vi "svl_Check Integration Time.vi"(4 "integration time":dbl=1.0 format="%.2f", 6 "acquisition period":dbl=1.0 format="%.2f", 8 "error in (no error)":errorcluster, 9 "restart averaging (F)":bool) -> (0 "error out":errorcluster, 1 "blocks to integrate":i32=1, 2 "parameter has changed":bool)   [LabVIEW 2017]
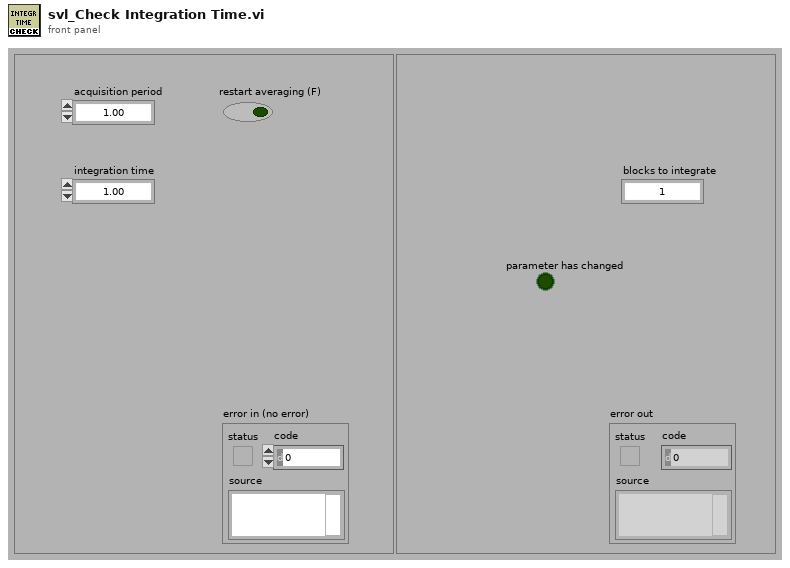
[diagram p1: front panel]
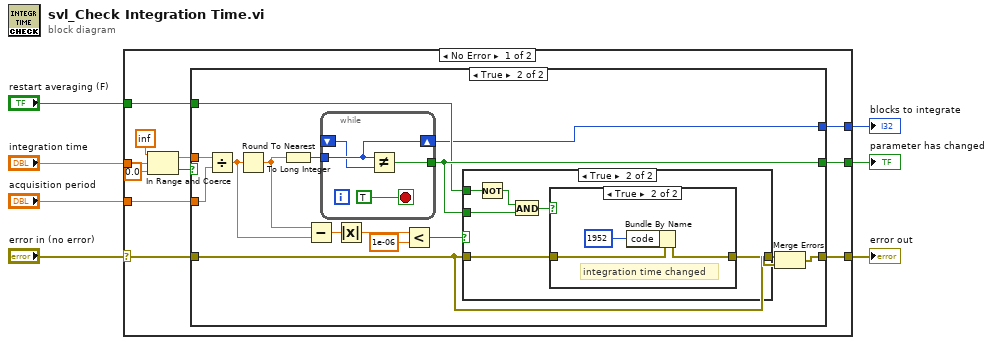
[diagram p0: block diagram]
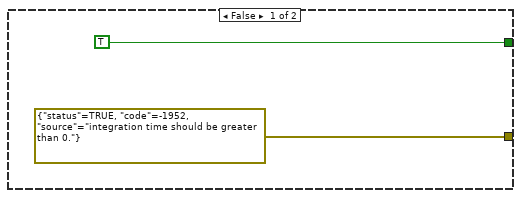
[diagram p2: hidden frame]
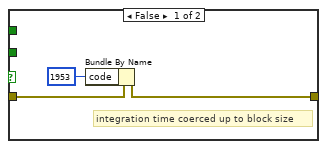
[diagram p3: hidden frame]
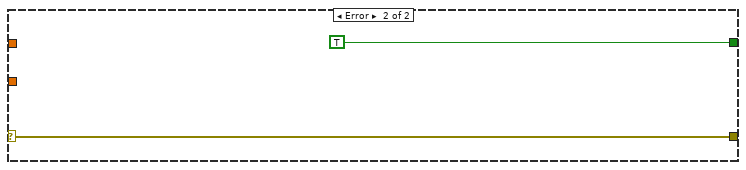
[diagram p5: hidden frame]
diagram:
  n1 = case shown="No Error" "error in (no error)" {
    selector: "error in (no error)" -> [w17 w53]
    tunnel: [w18 TRUE] -> w4
    tunnel: "integration time" -> [w14 _]
    tunnel: [w16 w53] -> w5
    tunnel: "acquisition period" -> [w15 _]
    tunnel: "restart averaging (F)" -> [w9 _]
    tunnel: [w8 _] -> w1
    frame No Error {
      n2 = In Range and Coerce(upper limit=inf, x=w14, lower limit=0.0) -> (coerced(x)=w13:dbl, In Range?=w10:bool)
      n3 = case shown="True" w10 {
        tunnel: [TRUE w35] -> w18
        tunnel: w13 -> [_ w34]
        tunnel: w17 -> [_ w21]
        tunnel: [errorcluster {"status"=TRUE, "code"=-1952, "source"="integration time should be greater than 0."} ("error IO") w22] -> w16
        tunnel: w15 -> [_ w33]
        tunnel: w9 -> [_ w30]
        tunnel: [_ w24] -> w8
        frame False {
        }
        frame True {
          n4 = Divide(x=w34, y=w33) -> (x/y=w31:dbl)
          n5 = Round To Nearest(number=w31) -> (nearest integer value=w26:dbl)
          n6 = To Long Integer(number=w26) -> (32bit integer=w25:i32)
          n7 = Subtract(x=w26, y=w31) -> (x-y=w32:dbl)
          n8 = while {
            tunnel: [w50] -> w35
            tunnel: w25 -> [w51]
            shift-left: _ -> [w49]
            shift-right: [w51] -> w24
            stop <- TRUE stop-if-true
            n9 = Not Equal?(x=w51, y=w49) -> (x != y?=w50:bool)
          }
          n10 = Absolute Value(x=w32) -> (abs(x)=w29:dbl)
          n11 = Less?(x=w29, y=1e-06 ("x")) -> (x < y?=w28:bool)
          n12 = case shown="True" w28 {
            tunnel: w35 -> [_ w42]
            tunnel: w21 -> [w38 w44]
            tunnel: [w36 w43] -> w23
            tunnel: w30 -> [_ w39]
            frame False {
              # "integration time coerced up to block size"
              n13 = Bundle By Name(cluster=w38, "code"=1953) -> (w36:errorcluster)
            }
            frame True {
              n14 = Not(x=w39) -> (.not. x?=w40:bool)
              n15 = And(x=w40, y=w42) -> (x .and. y?=w41:bool)
              n16 = case shown="True" w41 {
                tunnel: [w45 w46] -> w43
                tunnel: w44 -> [w45 w48]
                frame False {
                }
                frame True {
                  # "integration time changed"
                  n17 = Bundle By Name(cluster=w48, "code"=1952) -> (w46:errorcluster)
                }
              }
            }
          }
          n18 = Merge Errors(w21, w23) -> (w22:errorcluster)
        }
      }
    }
    frame Error {
    }
  }
  "parameter has changed" <- w4
  "error out" <- w5
  "blocks to integrate" <- w1
